vi "Minuteur_ScanPanel.vi"(8 "error in (no error)":errorcluster caption="entrée d'erreur (pas d'erreur)", 11 "Tools.lvclass":refnum<class "Tools.lvclass">) -> (0 "error out":errorcluster caption="sortie d'erreur", 3 "BaseDevice.lvclass Out":refnum<class "Tools.lvclass">)   [LabVIEW 2019, in "Tools.lvclass"]
uses:
  Tools.lvclass
  C:/Programmes Labview/LabScanV1A/DevicesClass/BaseDevice/BaseDevice.lvclass
  BaseDevice/ScanPos.ctl
panel:
  in  "UpdateScanTime":bool
  in  "MainProgQ":refnum<queue>
  in  "MainProgQEvent":refnum<user-event>
  in  "ModRap":bool caption="Modèle Rapide"
  out "Positions":dbl[](array[numeric])
  in  "Points":u32=1 caption="Max Sample Count" min=1 max=100000 step=1
  in  "Stop":bool
  out "Init Program":bool
  # "Minuteur"
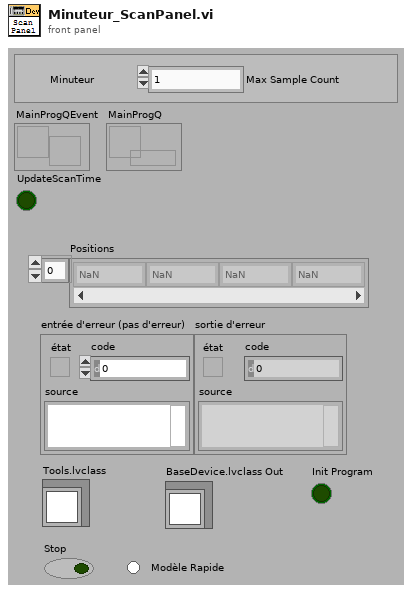
[diagram p1: front panel]
types:
  T1 = typedef "ScanPos.ctl" = cluster{"Debut":dbl, "Increment":dbl, "Fin":dbl, "Positions":dbl[], "Bidir":bool, "ModelRap":bool}
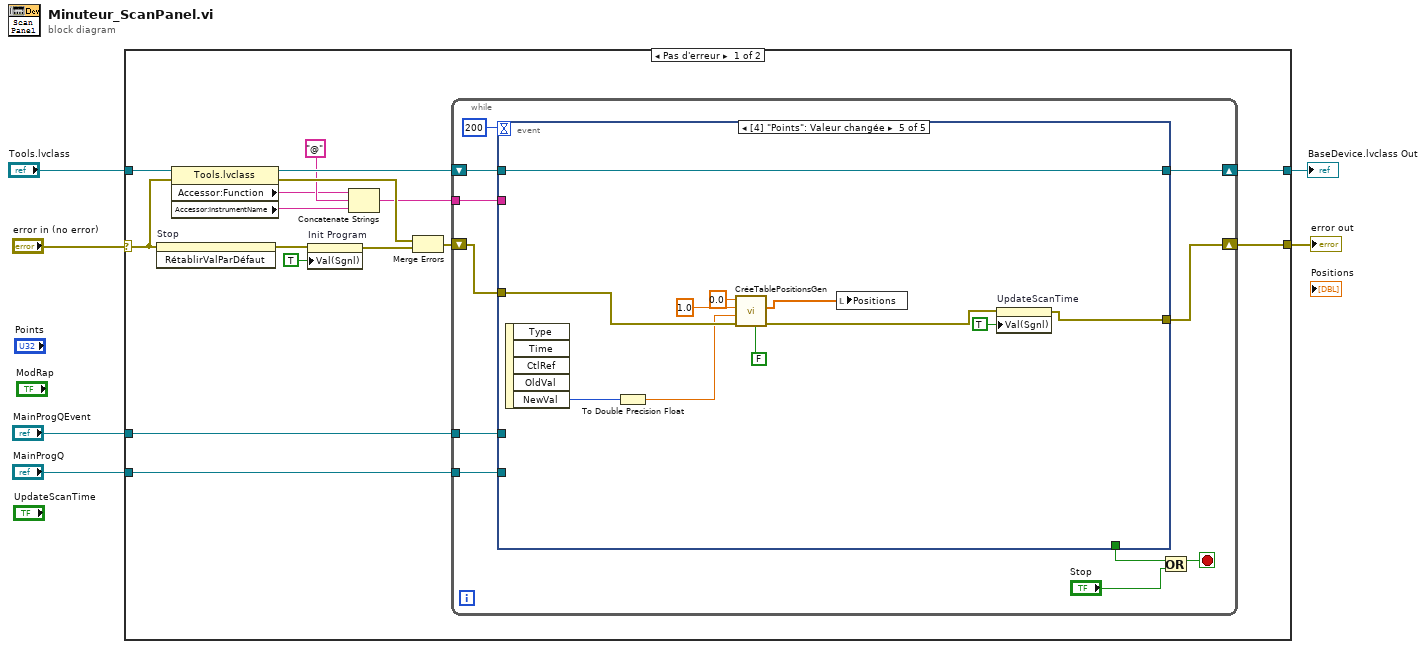
[diagram p0: block diagram]
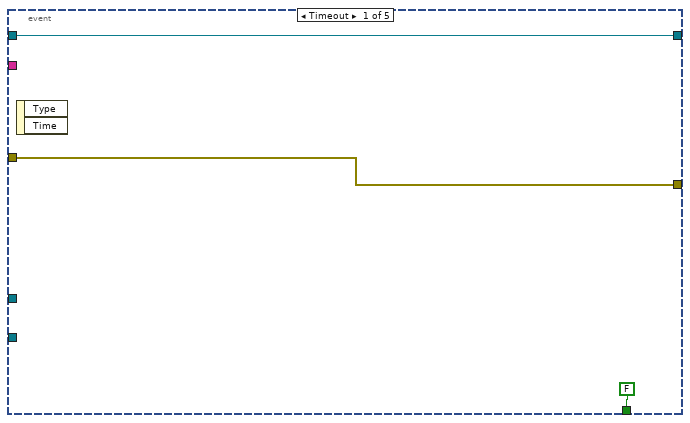
[diagram p2: hidden frame]
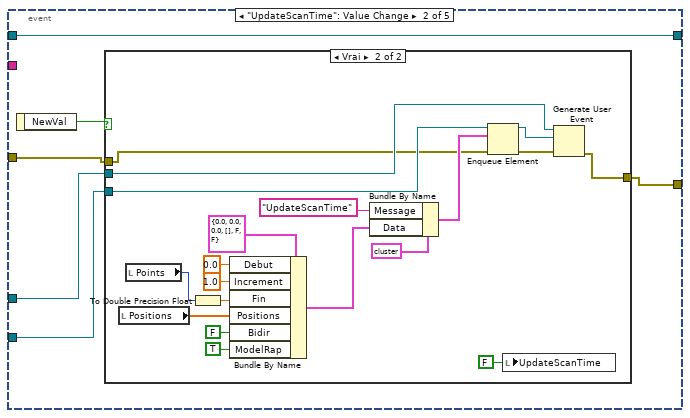
[diagram p3: hidden frame]
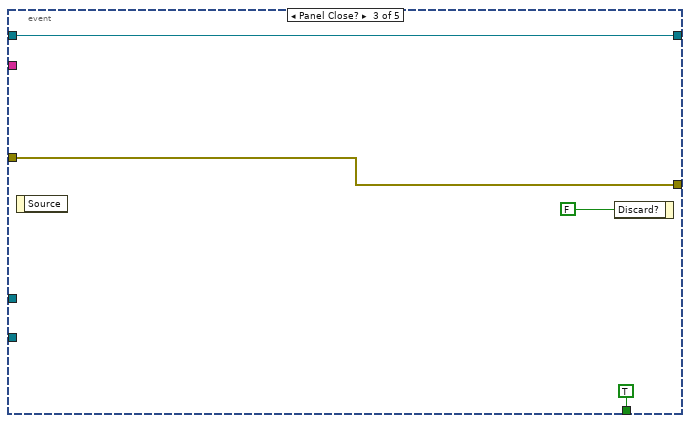
[diagram p5: hidden frame]
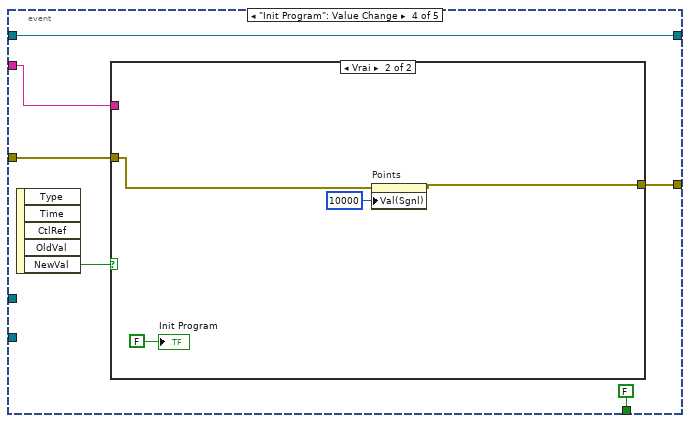
[diagram p6: hidden frame]
diagram:
  n1 = case shown="Pas d'erreur" "error in (no error)" {
    selector: "error in (no error)" -> [w16 w90]
    tunnel: [w22 w90] -> w5
    tunnel: "Tools.lvclass" -> [w21 w89]
    tunnel: [w19 w89] -> w3
    tunnel: "MainProgQEvent" -> [w8 _]
    tunnel: "MainProgQ" -> [w7 _]
    frame No Error {
      n2 = invoke on="Stop" class="Bool (strict)" method="RétablirValParDéfaut"(error in=w16) -> (error out=w18:errorcluster)  [unwired: 2 in, 2 out]
      n3 = property class="Tools.lvclass"(reference=w21, error in=w16) -> (reference out=w17:refnum<class "Tools.lvclass">, error out=w14:errorcluster, "Accessor:Function"=w11:string, "Accessor:InstrumentName"=w10:string)
      n4 = property on="Init Program" class="Bool (strict)"(error in=w18, "Val(Sgnl)"=TRUE ("Valeur (Signalisation)")) -> (error out=w15:errorcluster)  [unwired: 1 in, 1 out]
      n5 = Concatenate Strings(w11, "@" ("chaîne"), w10) -> (w9:string)
      n6 = Merge Errors(w14, w15) -> (w13:errorcluster)
      n7 = while {
        shift-right: [w32] -> w22
        shift-left: w13 -> [w25]
        shift-right: [w29] -> w19
        shift-left: w17 -> [w31]
        tunnel: w9 -> [w26]
        tunnel: w8 -> [w24]
        tunnel: w7 -> [w23]
        stop <- w28 stop-if-true
        n8 = event shown="[4] \"Points\": Valeur changée" {
          selector: _ -> [_ _ _ _ _]
          dyn-events: _ -> [_ _ _ _ _]
          timeout: 200 -> [_ _ _ _ _]
          tunnel: w25 -> [w34 w39 w64 w71 w84]
          tunnel: [w34 w37 w64 w70 w78] -> w32
          tunnel: w31 -> [w35 w38 w63 w69 w82]
          tunnel: [FALSE _ TRUE FALSE _] -> w30
          tunnel: [w35 w38 w63 w69 w82] -> w29
          tunnel: w26 -> [_ _ _ w67 _]
          tunnel: w24 -> [_ w42 _ _ _]
          tunnel: w23 -> [_ w41 _ _ _]
          event Timeout {
            n9 = event-data() -> ()  [unwired: 1 in, 2 out]
          }
          event "UpdateScanTime": Value Change {
            n10 = event-data() -> ("NewVal"=w40:bool)  [unwired: 1 in]
            n11 = case shown="Vrai" w40 {
              tunnel: w42 -> [_ w57]
              tunnel: w41 -> [_ w56]
              tunnel: [w43 w55] -> w37
              tunnel: w39 -> [w43 w50]
              frame False {
              }
              frame True {
                n12 = local read "Positions"() -> (w54:dbl[])
                n13 = local read "Points"() -> (w47:u32)
                n14 = To Double Precision Float(number=w47) -> (double precision float=w46:dbl)
                n15 = Bundle By Name(cluster=T1 {"Debut"=0.0, "Increment"=0.0, "Fin"=0.0, "Positions"=[], "Bidir"=FALSE, "ModelRap"=FALSE}, "Debut"=0.0, "Increment"=1.0, "Fin"=w46, "Positions"=w54, "Bidir"=FALSE, "ModelRap"=TRUE) -> (w52:T1)
                n16 = Bundle By Name(cluster=cluster{"Message":string, "Data":variant, i32} {"Message"="", "Data"=variant, 0} ("élément"), "Message"="UpdateScanTime", "Data"=w52) -> (w61:cluster{"Message":string, "Data":variant, i32})
                n17 = Enqueue Element(queue=w56, element=w61, error in (no error)=w50) -> (queue out=w60:refnum<queue>, error out=w59:errorcluster)  [unwired: 1 in, 1 out]
                n18 = local write "UpdateScanTime"(FALSE ("UpdateScanTime")) -> ()
                n19 = Generate User Event(user event=w57, event data cluster=w60, error in=w59) -> (error out=w55:errorcluster)  [unwired: 1 in, 1 out]
              }
            }
          }
          event Panel Close? {
            n20 = event-data() -> ()  [unwired: 1 in, 1 out]
            n21 = event-data("Discard?"=FALSE ("Rejeter ?")) -> ()  [unwired: 1 in, 1 out]
          }
          event "Init Program": Value Change {
            n22 = event-data() -> ("NewVal"=w72:bool)  [unwired: 1 in, 4 out]
            n23 = case shown="Vrai" w72 {
              tunnel: w67 -> [_ _]
              tunnel: w71 -> [w73 w76]
              tunnel: [w73 w74] -> w70
              frame False {
              }
              frame True {
                n24 = property on="Points" class="NumNb (strict)"(error in=w76, "Val(Sgnl)"=u32 10000 ("Value (Signaling)")) -> (error out=w74:errorcluster)  [unwired: 1 in, 1 out]
                "Init Program" <- FALSE
              }
            }
          }
          event "Points": Value Change {
            n25 = event-data() -> ("NewVal"=w86:u32)  [unwired: 1 in, 4 out]
            n26 = To Double Precision Float(number=w86) -> (double precision float=w81:dbl)
            n27 = call "CréeTablePositionsGen.vi"("IncFin (T)"=FALSE, "error in (no error)"=w84, "Fin"=w81, "Increment"=1.0, "Debut"=0.0) -> ("error out"=w79:errorcluster, "Positions"=w85:dbl[])  [unwired: 4 in, 1 out]
            n28 = local write "Positions"(w85) -> ()
            n29 = property on="UpdateScanTime" class="Bool (strict)"(error in=w79, "Val(Sgnl)"=TRUE ("Valeur (Signalisation)")) -> (error out=w78:errorcluster)  [unwired: 1 in, 1 out]
          }
        }
        n30 = Or(x=w30, y="Stop") -> (x .or. y?=w28:bool)
      }
    }
    frame Error {
    }
  }
  "error out" <- w5
  "BaseDevice.lvclass Out" <- w3
